vi "Launcher.vi"   [LabVIEW 2020]
uses:
  My First Actor.lvclass
  C:/Program Files (x86)/National Instruments/LabVIEW 2020/vi.lib/ActorFramework/Actor/Actor.lvclass
  My First Actor Messages/Popup Msg/Popup Msg.lvclass/Popup Msg.ctl
  <vilib>/ActorFramework/Message Enqueuer/Message Enqueuer.lvclass/Message Enqueuer.ctl
  <vilib>/ActorFramework/Message Enqueuer/Enqueue.vi
  My First Actor Messages/Popup Msg/Popup Msg.lvclass
  C:/Program Files (x86)/National Instruments/LabVIEW 2020/vi.lib/ActorFramework/Message/Message.lvclass
  <vilib>/ActorFramework/Stop Msg/Stop Msg.lvclass
  <vilib>/ActorFramework/Message Priority Queue/Priority Enqueue.vi
  <vilib>/ActorFramework/Actor/Actor.lvclass
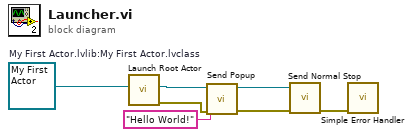
[diagram p0: block diagram]
diagram:
  w7 = refnum<class "My First Actor.lvclass"> refnum  # My First Actor.lvlib:My First Actor.lvclass
  n1 = call <vilib>:"Launch Root Actor.vi"("Actor"=w7) -> ("error out"=w1:errorcluster, "Actor's Enqueuer"=w6:refnum<class "Message Enqueuer.lvclass">)  [unwired: 9 in]
  n2 = call "Send Popup.vi"("error in (no error)"=w1, "String"="Hello World!", "Message Enqueuer"=w6) -> ("error out"=w2:errorcluster, "Message Enqueuer out"=w4:refnum<class "Message Enqueuer.lvclass">)  [unwired: 7 in]
  n3 = call <vilib>:"Send Normal Stop.vi"("error in (no error)"=w2, "Message Enqueuer"=w4) -> ("error out"=w3:errorcluster)  [unwired: 9 in]
  n4 = call <vilib>:"Simple Error Handler.vi"("error in (no error)"=w3) -> ()  [unwired: 4 in, 5 out]
